vi "Practica1_Comparador.vi"() -> ()   [LabVIEW 2015]
uses:
  <vilib>/LabVIEW Interface for Arduino/LabVIEW Interface for Arduino.lvlib
panel:
  in  "Desconectar":bool
  out "Medidor":dbl(knob) scale=0.0..5.0
  out "Menor que 2.5v":bool
  out "Mayor que 2.5v":bool
  out "Valor Leido":dbl(slide) scale=0.0..5.0
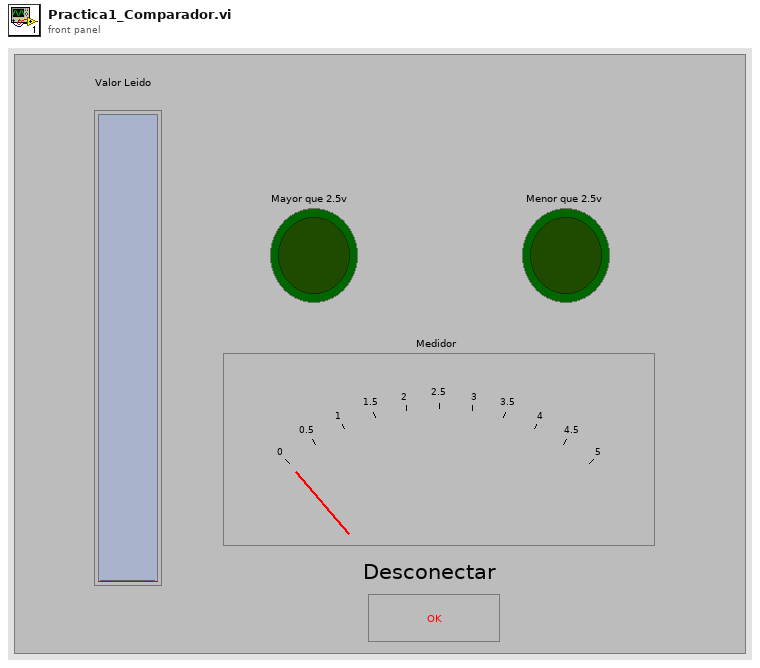
[diagram p1: front panel]
types:
  T1 = typedef "LabVIEW Interface for Arduino.lvlib/Arduino Resource.ctl" = cluster{"VISA resource":refnum<visa-resource-name>, "Board Type":T2, "Connection Type":enum8{"USB / Serial"}, "Bytes Per Packet (15)":u8}
  T2 = typedef "LabVIEW Interface for Arduino.lvlib/Board Type.ctl" = enum16{"Uno", "Dimuelanove w/Atmega 328", "Mega 2560"}
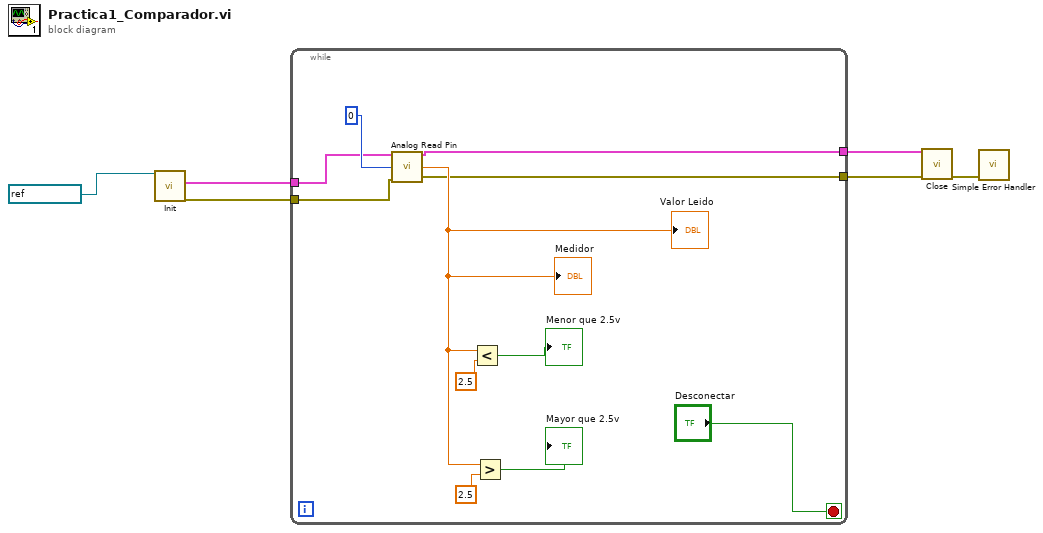
[diagram p0: block diagram]
diagram:
  n1 = call <vilib>:"Init.vi"("VISA resource"=refnum<visa-resource-name> "COM3") -> ("Arduino Resource"=w5:T1, "error out"=w4:errorcluster)  [unwired: 17 in]
  n2 = while {
    tunnel: w5 -> [w15]
    tunnel: w4 -> [w14]
    tunnel: [w8] -> w3
    tunnel: [w7] -> w2
    stop <- "Desconectar" stop-if-true
    n3 = call <vilib>:"Analog Read Pin.vi"("Arduino Resource"=w15, "Analog Input Pin (0)"=u8 0, "error in"=w14) -> ("Arduino Resource"=w8:T1, "Voltage"=w9:dbl, "error out"=w7:errorcluster)  [unwired: 10 in]
    "Medidor" <- w9
    "Valor Leido" <- w9
    n4 = Less?(x=w9, y=2.5) -> (x < y?=→"Menor que 2.5v":bool)
    n5 = Greater?(x=w9, y=2.5) -> (0:→"Mayor que 2.5v":bool)
  }
  n6 = call <vilib>:"Close.vi"("Arduino Resource"=w3, "error in"=w2) -> ("error out"=w1:errorcluster)  [unwired: 13 in]
  n7 = call <vilib>:"Simple Error Handler.vi"("error in (no error)"=w1) -> ()  [unwired: 4 in, 5 out]
